vi "Acquirer.vi"(11 "command stream":T1) -> (0 "wfm data stream":T4, 3 "file path tag":T5, 4 "status stream":T2, 6 "wfm data lossy stream":T3)   [LabVIEW 2019]
uses:
  <extravilib>/ChannelInstances/Tag-path/))Channel.ctl
  <extravilib>/ChannelInstances/Stream-a[.](wfm(dbl))/)Channel.ctl
  <extravilib>/ChannelInstances/Lossy Stream-a[.](wfm(dbl))/)Channel.ctl
  <extravilib>/ChannelInstances/Stream-str/)Channel.ctl
  <resource>/Channels/Messenger/))Channel.ctl
  <vilib>/ChannelSupport/Channel Message/Channel Message.lvclass
  messages/MeasureAndLogMessage.lvclass/MeasureAndLogMessage.ctl
  subVIs/Measure and Log Settings.ctl
  subVIs/Simulated Signal Type.ctl
  <resource>/Channels/Messenger/Read With Abort.vi
  <vilib>/ChannelSupport/Channel Message/Read ID.vi
  <extravilib>/ChannelInstances/Stream-a[.](wfm(dbl))/Endpoint.vi
  <extravilib>/ChannelInstances/Lossy Stream-a[.](wfm(dbl))/Endpoint.vi
  <extravilib>/ChannelInstances/Stream-str/Endpoint.vi
  <resource>/Channels/Messenger/Endpoint.vi
  <extravilib>/ChannelInstances/Tag-path/Endpoint.vi
  <extravilib>/ChannelInstances/Stream-a[.](wfm(dbl))/)Channel.vi
  <resource>/ChannelSupport/_ChannelSupport/WaitIfNeeded.vi
  <extravilib>/ChannelInstances/Lossy Stream-a[.](wfm(dbl))/)Channel.vi
  <extravilib>/ChannelInstances/Stream-str/)Channel.vi
  messages/MeasureAndLogMessage.lvclass
  <resource>/Channels/Messenger/Messenger.lvlib
  <extravilib>/ChannelInstances/Tag-path.lvlib
  <extravilib>/ChannelInstances/Stream-str.lvlib
  <extravilib>/ChannelInstances/Lossy Stream-a[.](wfm(dbl)).lvlib
  <extravilib>/ChannelInstances/Stream-a[.](wfm(dbl)).lvlib
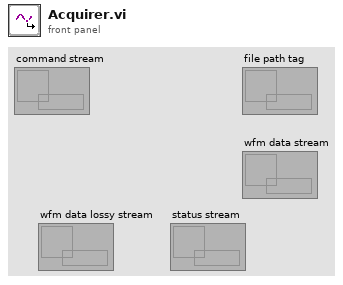
[diagram p1: front panel]
types:
  T1 = typedef "Messenger.lvlib/))Channel.ctl" = refnum<queue>
  T2 = typedef "Stream-str.lvlib/)Channel.ctl" = refnum<queue>
  T3 = typedef "Lossy Stream-a[.](wfm(dbl)).lvlib/)Channel.ctl" = refnum<queue>
  T4 = typedef "Stream-a[.](wfm(dbl)).lvlib/)Channel.ctl" = refnum<queue>
  T5 = typedef "Tag-path.lvlib/))Channel.ctl" = refnum<queue>
  T6 = typedef "Measure and Log Settings.ctl" = cluster{"sample rate":dbl, "input range":dbl, "logfile path":path, "Simulated Signal":cluster{"signal type":T7, "frequency":dbl, "amplitude":dbl}}
  T7 = typedef "Simulated Signal Type.ctl" = enum16{"Sine Wave", "Square Wave with Noise"}
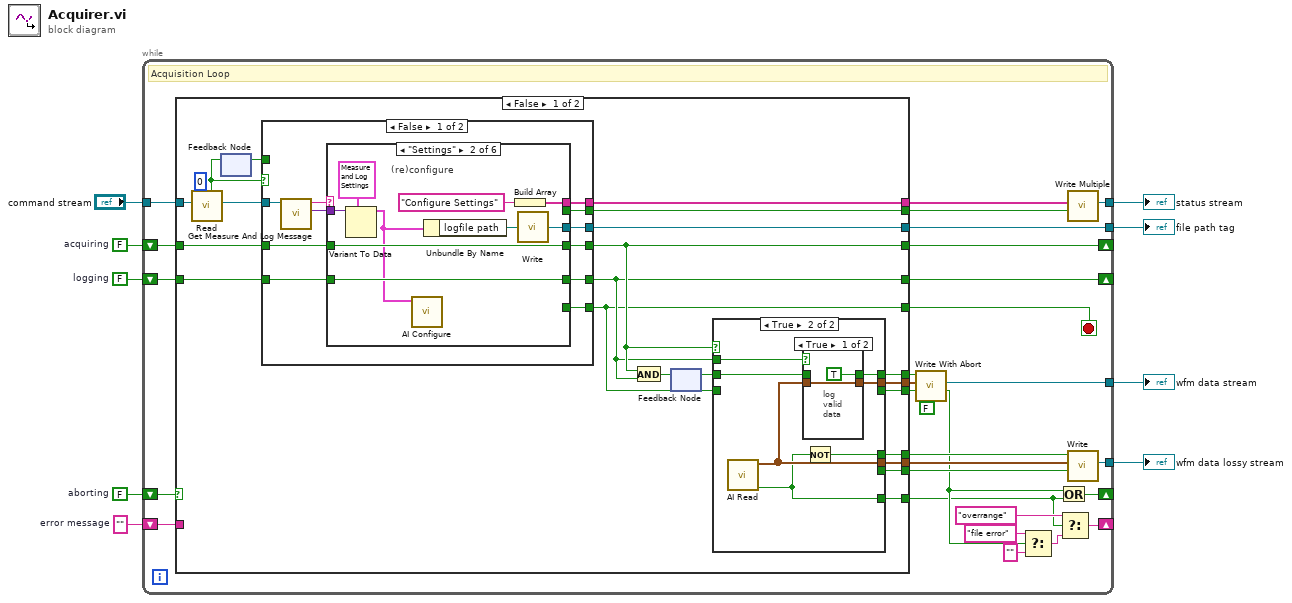
[diagram p0: block diagram]
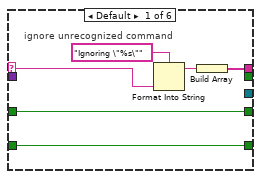
[diagram p2: hidden frame]
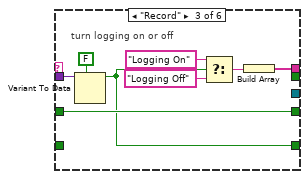
[diagram p3: hidden frame]
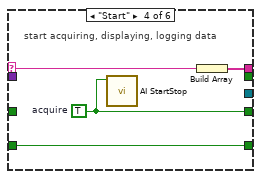
[diagram p4: hidden frame]
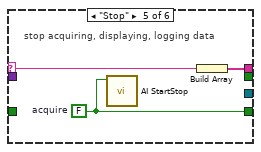
[diagram p5: hidden frame]
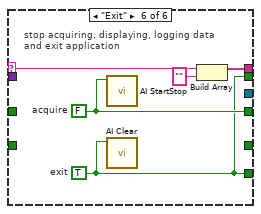
[diagram p6: hidden frame]
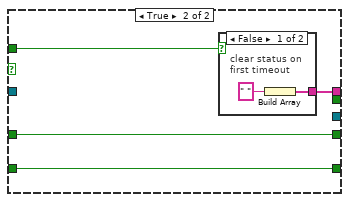
[diagram p7: hidden frame]
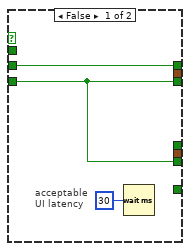
[diagram p9: hidden frame]
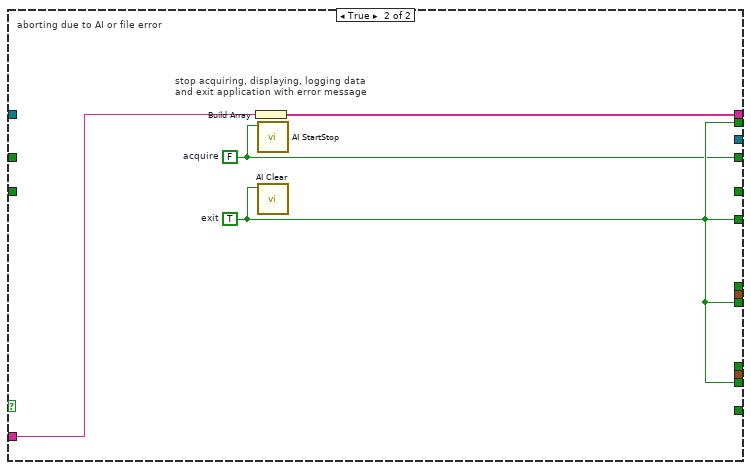
[diagram p11: hidden frame]
diagram:
  w5 = ""  # error message
  w4 = FALSE  # aborting
  w3 = FALSE  # logging
  w2 = FALSE  # acquiring
  n1 = while {
    tunnel: "command stream" -> [w37]
    tunnel: [w29] -> w6
    tunnel: [w26] -> w7
    tunnel: [w22] -> w8
    shift-right: [w34] -> _
    shift-left: w2 -> [w35]
    shift-right: [w33] -> _
    shift-left: w3 -> [w38]
    tunnel: [w36] -> w9
    shift-right: [w21] -> _
    shift-left: w4 -> [w32]
    shift-right: [w12] -> _
    shift-left: w5 -> [w31]
    stop <- w30 stop-if-true
    # "Acquisition Loop"
    n2 = case shown="False" w32 {
      tunnel: w38 -> [w60 _]
      tunnel: w37 -> [w59 _]
      tunnel: [w54 _] -> w36
      tunnel: w35 -> [w53 _]
      tunnel: [w52 w126] -> w34
      tunnel: [w51 _] -> w33
      tunnel: [w48 w127] -> w30
      tunnel: w31 -> [_ w129]
      tunnel: [w46 w127] -> w28
      tunnel: [w47 w128] -> w27
      tunnel: [w44 w127] -> w25
      tunnel: [w45 _] -> w24
      tunnel: [w43 _] -> w23
      tunnel: [w42 _] -> w13
      tunnel: [w41 _] -> w20
      tunnel: [w40 w127] -> w19
      tunnel: [w39 _] -> w18
      frame False {
        n3 = call <resource>:"Read.vi"("timeout in ms (-1)"=0, "channel"=w59) -> ("element"=w58:refnum<class "Channel Message.lvclass">, "timed out?"=w56:bool)  [unwired: 7 in, 1 out]
        n4 = feedback #1() -> (w55:bool)  [unwired: 1 in]
        n5 = feedback-in #1(w56) -> ()
        n6 = case shown="False" w56 {
          tunnel: w58 -> [w71 _]
          tunnel: [w68 _] -> w48
          tunnel: [w67 w110] -> w52
          tunnel: w53 -> [w66 w110]
          tunnel: [w65 w109] -> w51
          tunnel: w60 -> [w64 w109]
          tunnel: w55 -> [_ w108]
          tunnel: [w63 _] -> w54
          tunnel: [w62 w107] -> w47
          tunnel: [w61 _] -> w46
          frame False {
            n7 = call "Get Measure And Log Message.vi"("MyMessage"=w71) -> ("args"=w69:variant, "command"=w70:string)  [unwired: 7 in, 2 out]
            n8 = case shown="\"Settings\"" w70 {
              selector: w70 -> [w77 _ _ w96 w101 w106]
              tunnel: w69 -> [_ w84 w93 _ _ _]
              tunnel: [_ _ _ _ _ w102] -> w68
              tunnel: [w75 w86 w94 w98 w99 w103] -> w67
              tunnel: w66 -> [w75 w86 w94 _ _ _]
              tunnel: [w74 w85 w89 w97 _ _] -> w65
              tunnel: w64 -> [w74 w85 _ w97 _ _]
              tunnel: [_ w81 _ _ _ _] -> w63
              tunnel: [w72 w78 w87 w95 w100 w104] -> w62
              tunnel: [_ _ _ _ _ w102] -> w61
              frame Default {
                # "ignore unrecognized command"
                n9 = Format Into String(format string="Ignoring \"%s\"", w77) -> (resulting string=w73:string)  [unwired: 2 in, 1 out]
                n10 = Build Array(w73) -> (w72:string[])
              }
              frame "Settings" {
                # "(re)configure"
                n11 = Variant To Data(type=T6 {"sample rate"=100.0, "input range"=10.0, "logfile path"=path "/Bohr/Users/jeffk/Documents/LabVIEW Data/Logged Data.tdms", "Simulated Signal"={"signal type"=enum."Sine Wave", "frequency"=1000.0, "amplitude"=5.0}} ("settings out"), Variant=w84) -> (data=w83:T6)  [unwired: 1 in, 1 out]
                n12 = call "AI Configure.vi"("settings in"=w83) -> ()  [unwired: 11 in]
                n13 = Unbundle By Name(w83) -> ("logfile path"=w82:path)
                n14 = Build Array("Configure Settings" ("element")) -> (w78:string[])
                n15 = call <extravilib>:"Write.vi"("element"=w82) -> ("channel"=w81:T5)  [unwired: 1 out]
              }
              frame "Record" {
                # "turn logging on or off"
                n16 = Variant To Data(type=FALSE, Variant=w93) -> (data=w89:bool)  [unwired: 1 in, 1 out]
                n17 = Select(t="Logging On", s=w89, f="Logging Off") -> (s? t:f=w88:string)
                n18 = Build Array(w88) -> (w87:string[])
              }
              frame "Start" {
                w98 = TRUE  # acquire
                # "start acquiring, displaying, logging data"
                n19 = call "AI StartStop.vi"("acquire"=w98) -> ()  [unwired: 11 in]
                n20 = Build Array(w96) -> (w95:string[])
              }
              frame "Stop" {
                w99 = FALSE  # acquire
                # "stop acquiring, displaying, logging data"
                n21 = call "AI StartStop.vi"("acquire"=w99) -> ()  [unwired: 11 in]
                n22 = Build Array(w101) -> (w100:string[])
              }
              frame "Exit" {
                w103 = FALSE  # acquire
                w102 = TRUE  # exit
                # "stop acquiring, displaying, logging data\nand exit application"
                n23 = call "AI StartStop.vi"("acquire"=w103) -> ()  [unwired: 11 in]
                n24 = call "AI Clear.vi"("clear"=w102) -> ()  [unwired: 11 in]
                n25 = Build Array(w106, "" ("element")) -> (w104:string[])
              }
            }
          }
          frame True {
            n26 = case shown="False" w108 {
              tunnel: [w111 _] -> w107
              frame False {
                # "clear status on\nfirst timeout"
                n27 = Build Array(" " ("string")) -> (w111:string[])
              }
              frame True {
              }
            }
          }
        }
        n28 = And(x=w52, y=w51) -> (x .and. y?=w50:bool)
        n29 = feedback #2() -> (w49:bool)  [unwired: 1 in]
        n30 = feedback-in #2(w50) -> ()
        n31 = case shown="True" w52 {
          tunnel: w51 -> [_ w122]
          tunnel: w49 -> [w115 w121]
          tunnel: w48 -> [w114 _]
          tunnel: [_ w120] -> w45
          tunnel: [w114 _] -> w44
          tunnel: [_ w117] -> w43
          tunnel: [_ w116] -> w42
          tunnel: [w115 w118] -> w41
          tunnel: [w114 _] -> w40
          tunnel: [_ w119] -> w39
          frame False {
            # "acceptable\nUI latency"
            n32 = Wait (ms)(milliseconds to wait=u32 30) -> ()  [unwired: 1 out]
          }
          frame True {
            n33 = call "AI Read.vi"() -> ("error"=w116:bool, "waveforms"=w117:waveform(dbl)[])  [unwired: 10 in]
            n34 = case shown="True" w122 {
              tunnel: w117 -> [w124 _]
              tunnel: w121 -> [_ w125]
              tunnel: [w124 _] -> w119
              tunnel: [TRUE w125] -> w118
              frame True {
                # "log \nvalid\ndata"
              }
              frame False {
              }
            }
            n35 = Not(x=w116) -> (.not. x?=w120:bool)
          }
        }
      }
      frame True {
        w126 = FALSE  # acquire
        w127 = TRUE  # exit
        # "aborting due to AI or file error"
        # "stop acquiring, displaying, logging data\nand exit application with error message"
        n36 = Build Array(w129) -> (w128:string[])
        n37 = call "AI StartStop.vi"("acquire"=w126) -> ()  [unwired: 11 in]
        n38 = call "AI Clear.vi"("clear"=w127) -> ()  [unwired: 11 in]
      }
    }
    n39 = call <extravilib>:"Write With Abort.vi"("abort"=FALSE, "last element? (F)"=w19, "element"=w18, "element valid? (T)"=w20) -> ("aborted?"=w16:bool, "channel"=w22:T4)  [unwired: 4 in, 2 out]
    n40 = Select(t="file error", s=w16, f="") -> (s? t:f=w11:string)
    n41 = Or(x=w16, y=w13) -> (x .or. y?=w21:bool)
    n42 = Select(t="overrange", s=w13, f=w11) -> (s? t:f=w12:string)
    n43 = call <extravilib>:"Write Multiple.vi"("last element? (F)"=w28, "elements"=w27) -> ("channel"=w29:T2)  [unwired: 6 in, 3 out]
    n44 = call <extravilib>:"Write.vi"("last element? (F)"=w25, "element"=w23, "element valid? (T)"=w24) -> ("channel"=w26:T3)  [unwired: 6 in, 2 out]
  }
  "file path tag" <- w9
  "wfm data stream" <- w8
  "wfm data lossy stream" <- w7
  "status stream" <- w6
